vi "Read Cell Status File.vi"(0 "FilePathIn":path=path "C:/ER2007/Cell Status.dat", 1 "Cell Select":i32=8) -> (4 "P-Xdcr":enum16{"<none>", "Lo Range", "Hi Range"}[](array[ring]), 5 "Pdn":dbl[](array[numeric]) format="%.1f", 6 "Pdp":dbl[](array[numeric]) format="%.1f", 7 "Next Time":dbl[](array[numeric]) format="%.1f", 8 "Run Status":bool[](array[boolean]), 9 "Elapsed-T":dbl[](array[numeric]) format="%.1f", 11 "Last_T":timestamp[](array[timestamp]) format="%<%H:%M>T", 12 "SampID":string[](array[string]), 13 "Last Resistor":T1(array[ring]), 14 "ER 1-2":dbl[](array[numeric]) format="%.3f", 15 "Pv":dbl[](array[numeric]) format="%.1f", 16 "ER 1-3":dbl[](array[numeric]) format="%.3f", 17 "Pp":dbl[](array[numeric]) format="%.1f", 18 "ER 1-4":dbl[](array[numeric]) format="%.3f", 19 "Pc":dbl[](array[numeric]) format="%.1f", 20 "FilePathOut":path=path "C:/ER2006/Cell Status.dat", 21 "Test Info":T3 {"Cell Data"."Rw Temp" format="%.2f"; "Cell Data"."Rw" format="%.2f"; "Cell Data"."DAQ Units" items=["Mins", "Hrs"]; "Cell Data"."CurData" format="%.3f"; "Cell Data"."Last Pore Vol" format="%.3f"; "Cell Data"."Amplitude" format="%.3f"; "Cell Data"."ElectSpace" format="%.2f"; "Cell Data"."Permeability" format="%.2f"; "Cell Data"."Porosity" format="%.2f"; "Cell Data"."Diameter" format="%.2f"; "Cell Data"."Length" format="%.2f"}, 22 "GenInfoOut":T2, 23 "ER 2-3":dbl[](array[numeric]) format="%.3f", 24 "F 2-3":dbl[](array[numeric]) format="%.3f", 25 "TA":dbl[](array[numeric]) format="%.1f", 26 "TB":dbl[](array[numeric]) format="%.1f", 27 "ErrorOut":errorcluster)   [LabVIEW 2013]
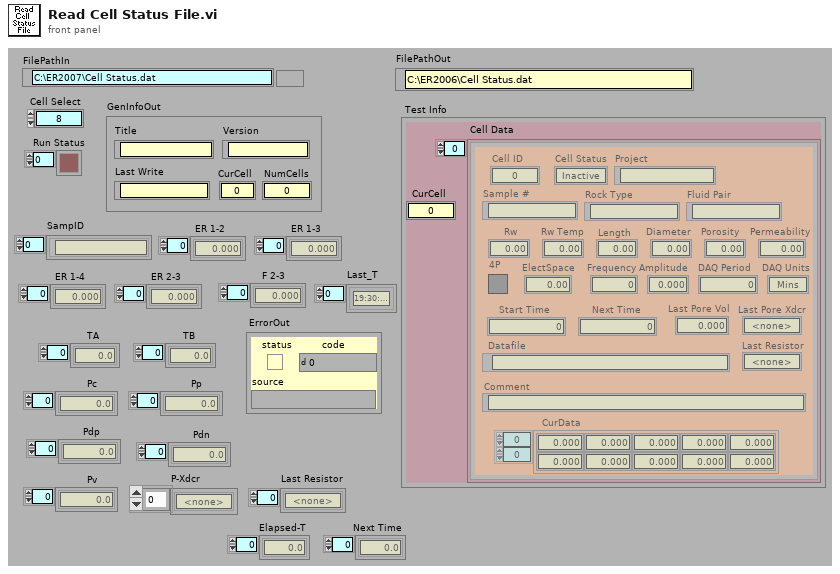
[diagram p1: front panel]
types:
  T1 = enum16{"<none>", "Resistor 1", "Resistor 2", "Resistor 3", "Resistor 4", "Resistor 5", "Resistor 6"}[]
  T2 = cluster{"Title":string, "Version":string, "Last Write":string, "CurCell":i32, "NumCells":i32}
  T3 = cluster{"CurCell":i32, "Cell Data":cluster{"Cell ID":i32, "Cell Status":enum16{"Inactive", "Setup", "Active", "Done"}, "Project":string, "Sample #":string, "Rock Type":string, "Fluid Pair":string, "Rw":dbl, "Rw Temp":dbl, "Length":dbl, "Diameter":dbl, "Porosity":dbl, "Permeability":dbl, "4P":bool, "ElectSpace":dbl, "Frequency":dbl, "Amplitude":dbl, "DAQ Period":u32, "DAQ Units":u16, "Start Time":dbl, "Next Time":dbl, "Datafile":path, "Last Pore Vol":dbl, "Last Pore Xdcr":enum16{"<none>", "Lo Range", "Hi Range"}, "Last Resistor":enum16{"<none>", "Resistor 1", "Resistor 2", "Resistor 3", "Resistor 4", "Resistor 5", "Resistor 6"}, "CurData":dbl[][], "Comment":string}[]}
  T4 = enum16{"New File", "Read Cell Status", "Write Cell Status"}
  T5 = cluster{"Cell ID":i32, "Cell Status":enum16{"Inactive", "Setup", "Active", "Done"}, "Project":string, "Sample #":string, "Rock Type":string, "Fluid Pair":string, "Rw":dbl, "Rw Temp":dbl, "Length":dbl, "Diameter":dbl, "Porosity":dbl, "Permeability":dbl, "4P":bool, "ElectSpace":dbl, "Frequency":dbl, "Amplitude":dbl, "DAQ Period":u32, "DAQ Units":u16, "Start Time":dbl, "Next Time":dbl, "Datafile":path, "Last Pore Vol":dbl, "Last Pore Xdcr":enum16{"<none>", "Lo Range", "Hi Range"}, "Last Resistor":enum16{"<none>", "Resistor 1", "Resistor 2", "Resistor 3", "Resistor 4", "Resistor 5", "Resistor 6"}, "CurData":dbl[][], "Comment":string}
  T6 = enum16{"<none>", "Resistor 1", "Resistor 2", "Resistor 3", "Resistor 4", "Resistor 5", "Resistor 6"}
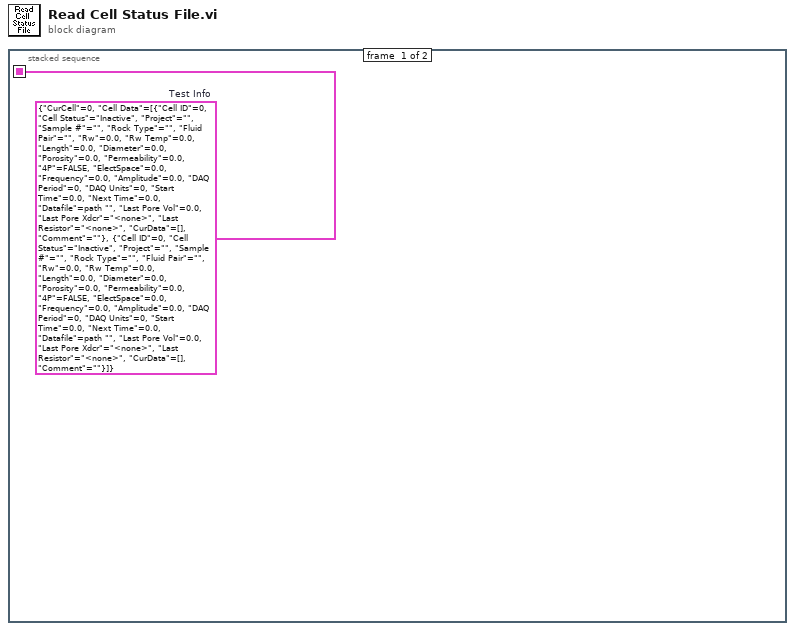
[diagram p0: block diagram]
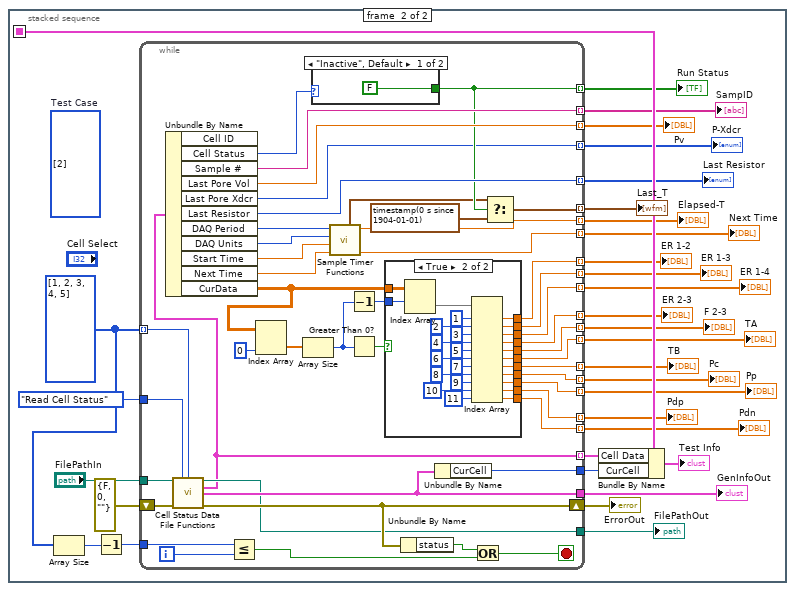
[diagram p2: hidden frame]
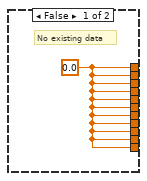
[diagram p3: hidden frame]
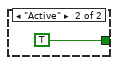
[diagram p4: hidden frame]
diagram:
  n1 = stacked-sequence {
    seq-local: [w1 _] -> [_ w27]
    frame #0 {
      w1 = T3 {"CurCell"=0, "Cell Data"=[{"Cell ID"=0, "Cell Status"=enum."Inactive", "Project"="", "Sample #"="", "Rock Type"="", "Fluid Pair"="", "Rw"=0.0, "Rw Temp"=0.0, "Length"=0.0, "Diameter"=0.0, "Porosity"=0.0, "Permeability"=0.0, "4P"=FALSE, "ElectSpace"=0.0, "Frequency"=0.0, "Amplitude"=0.0, "DAQ Period"=0, "DAQ Units"=0, "Start Time"=0.0, "Next Time"=0.0, "Datafile"=path "", "Last Pore Vol"=0.0, "Last Pore Xdcr"=enum."<none>", "Last Resistor"=enum."<none>", "CurData"=[], "Comment"=""}, {"Cell ID"=0, "Cell Status"=enum."Inactive", "Project"="", "Sample #"="", "Rock Type"="", "Fluid Pair"="", "Rw"=0.0, "Rw Temp"=0.0, "Length"=0.0, "Diameter"=0.0, "Porosity"=0.0, "Permeability"=0.0, "4P"=FALSE, "ElectSpace"=0.0, "Frequency"=0.0, "Amplitude"=0.0, "DAQ Period"=0, "DAQ Units"=0, "Start Time"=0.0, "Next Time"=0.0, "Datafile"=path "", "Last Pore Vol"=0.0, "Last Pore Xdcr"=enum."<none>", "Last Resistor"=enum."<none>", "CurData"=[], "Comment"=""}]}  # Test Info
    }
    frame #1 {
      (unwired) i32[] [2]  # Test Case
      w4 = i32[] [1, 2, 3, 4, 5]
      n2 = Array Size(array=w4) -> (size(s)=w30:i32)
      n3 = Decrement(x=w30) -> (x-1=w29:i32)
      n4 = while {
        tunnel: T4."Read Cell Status" ("Function") -> [w79]
        tunnel: "FilePathIn" -> [w78]
        tunnel: w4 -> [w47] mode=indexing
        shift-right: [w72] -> w23
        shift-left: errorcluster {"status"=FALSE, "code"=0, "source"=""} ("ErrorOut") -> [w77]
        tunnel: w29 -> [w76]
        tunnel: [w46] -> w26 mode=indexing
        tunnel: [w74] -> w28
        tunnel: [w73] -> w25
        tunnel: [w45] -> w24 mode=indexing
        tunnel: [w67] -> w22 mode=indexing
        tunnel: [w65] -> w21 mode=indexing
        tunnel: [w64] -> w20 mode=indexing
        tunnel: [w63] -> w19 mode=indexing
        tunnel: [w62] -> w18 mode=indexing
        tunnel: [w61] -> w17 mode=indexing
        tunnel: [w60] -> w16 mode=indexing
        tunnel: [w59] -> w15 mode=indexing
        tunnel: [w58] -> w14 mode=indexing
        tunnel: [w57] -> w13 mode=indexing
        tunnel: [w56] -> w12 mode=indexing
        tunnel: [w43] -> w11 mode=indexing
        tunnel: [w51] -> w10 mode=indexing
        tunnel: [w50] -> w9 mode=indexing
        tunnel: [w49] -> w8
        tunnel: [w48] -> w7 mode=indexing
        tunnel: [w37] -> w6 mode=indexing
        tunnel: [w36] -> w5 mode=indexing
        tunnel: [w34] -> w2 mode=indexing
        i -> [w75]
        stop <- w70 stop-if-true
        n5 = call "Cell Status Data File Functions.vi"("FilePathIn"=w78, "Function"=w79, "Cell Select - RO"=w47, "ErrorIn"=w77) -> ("FilePathOut"=w49:path, "Cell x Data Out"=w46:T5, "GenInfoOut"=w74:T2, "ErrorOut"=w72:errorcluster)  [unwired: 7 in, 1 out]
        n6 = Unbundle By Name(w46) -> ("Cell Status"=w68:enum16{"Inactive", "Setup", "Active", "Done"}, "Sample #"=w67:string, "Last Pore Vol"=w65:dbl, "Last Pore Xdcr"=w34:enum16{"<none>", "Lo Range", "Hi Range"}, "Last Resistor"=w48:T6, "DAQ Period"=w55:u32, "DAQ Units"=w54:u16, "Start Time"=w53:dbl, "Next Time"=w52:dbl, "CurData"=w40:dbl[][])  [unwired: 1 out]
        n7 = Less Or Equal?(x=w76, y=w75) -> (x <= y?=w71:bool)
        n8 = Index Array(array=w40, index (col)=0 ("disabled index (col)")) -> (element=w39:dbl[])  [unwired: 1 in]
        n9 = Array Size(array=w39) -> (size(s)=w35:i32)
        n10 = case shown="\"Inactive\", Default" w68 {
          tunnel: [FALSE TRUE] -> w45
          frame "Inactive", Default {
          }
          frame "Active" {
          }
        }
        n11 = call "Sample Timer Functions.vi"("Next Time In"=w52, "Start Time"=w53, "DAQ Units"=w54, "DAQ Period"=w55) -> ("Next Time Out"=w50:dbl, "Elapsed Hours"=w51:dbl, "Time"=w44:timestamp)  [unwired: 2 in, 3 out]
        n12 = Decrement(x=w35) -> (x-1=w66:i32)
        n13 = Greater Than 0?(x=w35) -> (x > 0?=w38:bool)
        n14 = case shown="True" w38 {
          tunnel: w66 -> [_ w105]
          tunnel: [w80 w103] -> w64
          tunnel: [w80 w101] -> w63
          tunnel: [w80 w99] -> w62
          tunnel: [w80 w97] -> w61
          tunnel: [w80 w95] -> w60
          tunnel: [w80 w93] -> w59
          tunnel: [w80 w91] -> w58
          tunnel: [w80 w89] -> w57
          tunnel: [w80 w87] -> w56
          tunnel: w40 -> [_ w85]
          tunnel: [w80 w82] -> w37
          tunnel: [w80 w81] -> w36
          frame False {
            w80 = 0.0 ("Numeric")
            # "No existing data"
          }
          frame True {
            n15 = Index Array(array=w85, index (row)=w105) -> (element=w104:dbl[])  [unwired: 1 in]
            n16 = Index Array(array=w104, index #1=1 ("index"), index #2=2 ("index"), index #3=3 ("index"), index #4=4 ("index"), index #5=5 ("index"), index #6=6 ("index"), index #7=7 ("index"), index #8=8 ("index"), index #9=9 ("index"), index #10=10 ("index"), index #11=11 ("index")) -> (element #1=w103:dbl, element #2=w101:dbl, element #3=w99:dbl, element #4=w97:dbl, element #5=w95:dbl, element #6=w93:dbl, element #7=w91:dbl, element #8=w89:dbl, element #9=w87:dbl, element #10=w82:dbl, element #11=w81:dbl)
          }
        }
        n17 = Unbundle By Name(w72) -> ("status"=w69:bool)
        n18 = Unbundle By Name(w74) -> ("CurCell"=w73:i32)
        n19 = Or(x=w69, y=w71) -> (x .or. y?=w70:bool)
        n20 = Select(t=w44, s=w45, f=timestamp(0 s since 1904-01-01)) -> (s? t:f=w43:timestamp)
      }
      "ErrorOut" <- w23
      "GenInfoOut" <- w28
      "Run Status" <- w24
      "SampID" <- w22
      "ER 1-3" <- w19
      "ER 1-4" <- w18
      "ER 2-3" <- w17
      "TA" <- w15
      "TB" <- w14
      "Pc" <- w13
      "Pp" <- w12
      "Pv" <- w21
      "Elapsed-T" <- w10
      "F 2-3" <- w16
      "ER 1-2" <- w20
      "Last_T" <- w11
      "FilePathOut" <- w8
      "Next Time" <- w9
      "Last Resistor" <- w7
      "Pdn" <- w5
      "Pdp" <- w6
      "P-Xdcr" <- w2
      n21 = Bundle By Name(cluster=w27, "Cell Data"=w26, "CurCell"=w25) -> (→"Test Info":T3)
    }
  }
